vi "generate_heap_and_hill_coordinates_1.vi"(8 "error in (no error)":errorcluster, 10 "ants":refnum<class "ant_base.lvclass">[](array[class])) -> (0 "error out":errorcluster, 1 "hillsArray":T5[](array[typedef]), 2 "foodHeapsArray":T1[](array[typedef])=[{"centerCoordinates"={"X"=100, "Y"=100}, "radius"=20.0, "volume"=1000, "Color"=5876991}, {"centerCoordinates"={"X"=140, "Y"=240}, "radius"=10.0, "volume"=10, "Color"=0}])   [LabVIEW 2015, in "world.lvlib" / "world.lvclass"]
doc: "generate coordinates of hills and heaps\nCreated by Artem Shevelev\nshevelev.pro\nartem@shevelev.pro\nLabVIEW Portal: https://labviewportal.org/memberlist.php?mode=viewprofile&u=2340"
uses:
  world.lvclass
  typedefs/worldPoint.ctl
  world.lvlib
  typedefs/worldPoint_cluster.ctl
  typedefs/anthill_cluster.ctl
  typedefs/foodHeap_cluster.ctl
  ant_base/ant_base.lvclass
  typedefs/amountOfFood.ctl
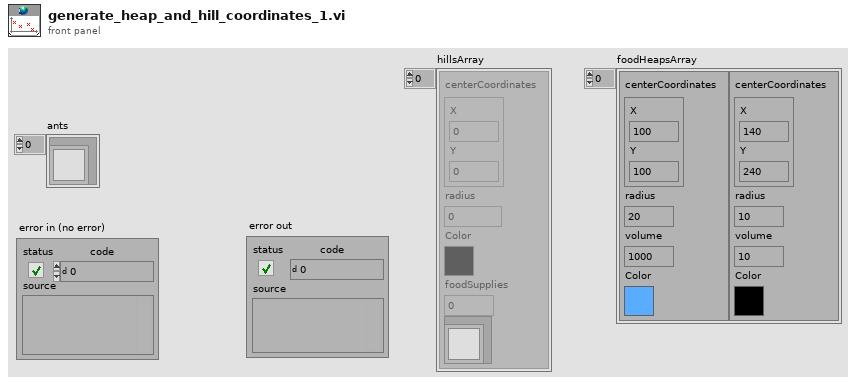
[diagram p1: front panel]
types:
  T1 = typedef "world.lvlib/foodHeap_cluster.ctl" = cluster{"centerCoordinates":T2, "radius":dbl, "volume":T4, "Color":u32}
  T2 = typedef "world.lvlib/worldPoint_cluster.ctl" = cluster{"X":T3, "Y":T3}
  T3 = typedef "world.lvlib/worldPoint.ctl" = i16
  T4 = typedef "world.lvlib/amountOfFood.ctl" = i32
  T5 = typedef "world.lvlib/anthill_cluster.ctl" = cluster{"centerCoordinates":T2, "radius":dbl, "Color":u32, "foodSupplies":T4, "antType":refnum<class "ant_base.lvclass">}
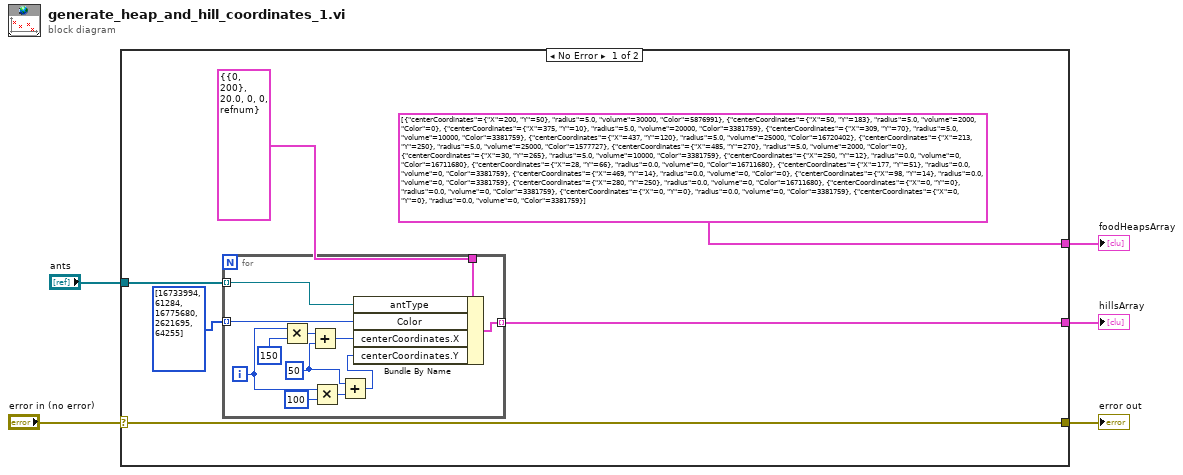
[diagram p0: block diagram]
diagram:
  n1 = case shown="No Error" "error in (no error)" {
    selector: "error in (no error)" -> [w8 w24]
    tunnel: [w9 _] -> w5
    tunnel: [T1[] [{"centerCoordinates"={"X"=200, "Y"=50}, "radius"=5.0, "volume"=30000, "Color"=5876991}, {"centerCoordinates"={"X"=50, "Y"=183}, "radius"=5.0, "volume"=2000, "Color"=0}, {"centerCoordinates"={"X"=375, "Y"=10}, "radius"=5.0, "volume"=20000, "Color"=3381759}, {"centerCoordinates"={"X"=309, "Y"=70}, "radius"=5.0, "volume"=10000, "Color"=3381759}, {"centerCoordinates"={"X"=437, "Y"=120}, "radius"=5.0, "volume"=25000, "Color"=16720402}, {"centerCoordinates"={"X"=213, "Y"=250}, "radius"=5.0, "volume"=25000, "Color"=1577727}, {"centerCoordinates"={"X"=485, "Y"=270}, "radius"=5.0, "volume"=2000, "Color"=0}, {"centerCoordinates"={"X"=30, "Y"=265}, "radius"=5.0, "volume"=10000, "Color"=3381759}, {"centerCoordinates"={"X"=250, "Y"=12}, "radius"=0.0, "volume"=0, "Color"=16711680}, {"centerCoordinates"={"X"=28, "Y"=66}, "radius"=0.0, "volume"=0, "Color"=16711680}, {"centerCoordinates"={"X"=177, "Y"=51}, "radius"=0.0, "volume"=0, "Color"=3381759}, {"centerCoordinates"={"X"=469, "Y"=14}, "radius"=0.0, "volume"=0, "Color"=0}, {"centerCoordinates"={"X"=98, "Y"=14}, "radius"=0.0, "volume"=0, "Color"=3381759}, {"centerCoordinates"={"X"=280, "Y"=250}, "radius"=0.0, "volume"=0, "Color"=16711680}, {"centerCoordinates"={"X"=0, "Y"=0}, "radius"=0.0, "volume"=0, "Color"=3381759}, {"centerCoordinates"={"X"=0, "Y"=0}, "radius"=0.0, "volume"=0, "Color"=3381759}, {"centerCoordinates"={"X"=0, "Y"=0}, "radius"=0.0, "volume"=0, "Color"=3381759}] ("foodHeapsArray") _] -> w4
    tunnel: [w8 w24] -> w2
    tunnel: "ants" -> [w7 _]
    frame No Error {
      n2 = for {
        tunnel: T5 {"centerCoordinates"={"X"=0, "Y"=200}, "radius"=20.0, "Color"=0, "foodSupplies"=0, "antType"=refnum} ("anthill") -> [w23]
        tunnel: u32[] [16733994, 61284, 16775680, 2621695, 64255] ("Color") -> [w22] mode=indexing
        tunnel: [w19] -> w9 mode=indexing
        tunnel: w7 -> [w18] mode=indexing
        i -> [w16]
        w13 = 50 ("y")
        n3 = Multiply(x=w16, y=150) -> (x*y=w21:i32)
        n4 = Add(x=w21, y=w13) -> (x+y=w17:i32)
        n5 = Multiply(x=w16, y=100) -> (x*y=w14:i32)
        n6 = Add(x=w13, y=w14) -> (x+y=w12:i32)
        n7 = Bundle By Name(cluster=w23, "antType"=w18, "Color"=w22, "centerCoordinates.X"=w17, "centerCoordinates.Y"=w12) -> (w19:T5)
      }
    }
    frame Error {
    }
  }
  "error out" <- w2
  "hillsArray" <- w5
  "foodHeapsArray" <- w4
